vi "rad_IP Address Validity Check.vi"(3 "IP Address":string) -> (1 "Valid IP":bool)   [LabVIEW 2020]
uses:
  <vilib>/regexp/Match Regular Expression.xnode
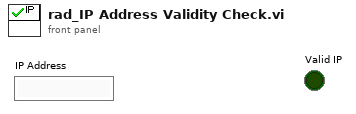
[diagram p1: front panel]
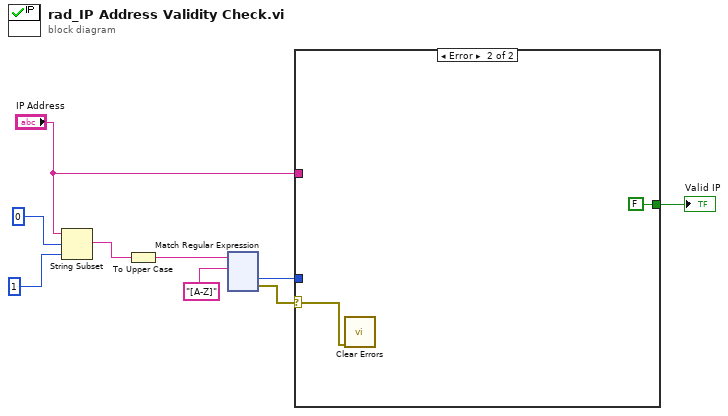
[diagram p0: block diagram]
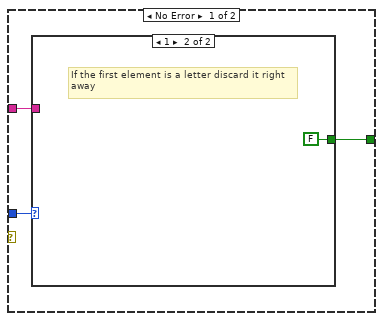
[diagram p2: hidden frame]
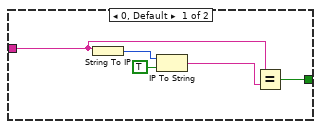
[diagram p3: hidden frame]
diagram:
  n1 = String Subset(string="IP Address", offset (0)=0, length (rest)=1 ("length (rest)")) -> (substring=w5:string)
  n2 = To Upper Case(1:w5) -> (0:w4:string)
  n3 = xnode "Match Regular Expression"("input string"=w4, "regular expression"="[A-Z]") -> ("offset past match"=w2:i32, "error out"=w1:errorcluster)  [unwired: 4 in, 3 out]
  n4 = case shown="Error" w1 {
    selector: w1 -> [_ w20]
    tunnel: "IP Address" -> [w12 _]
    tunnel: [w11 FALSE] -> w3
    tunnel: w2 -> [w10 _]
    frame No Error {
      n5 = case shown="1" w10 {
        tunnel: w12 -> [w17 _]
        tunnel: [w13 FALSE] -> w11
        frame 0, Default {
          n6 = String To IP(1:w17) -> (0:w16:u32)
          n7 = IP To String(1:TRUE ("dot notation? (F)"), 2:w16) -> (0:w14:string)
          n8 = Equal?(x=w17, y=w14) -> (x = y?=w13:bool)
        }
        frame 1 {
          # "If the first element is a letter discard it right\naway"
        }
      }
    }
    frame Error {
      n9 = call <vilib>:"Clear Errors.vi"("error in (no error)"=w20) -> ()  [unwired: 5 in, 2 out]
    }
  }
  "Valid IP" <- w3
